vi "Clear Tree.vi"(7 "Tree Refnum In":refnum<vi>, 8 "error in (no error)":errorcluster, 9 "Parent Tag In":string, 10 "Tree":string(tree), 11 "Clear Tree?":bool) -> (0 "error out":errorcluster, 1 "Parent Tag Out":string, 5 "Tree Refnum Out":refnum<vi>)   [LabVIEW 2023]
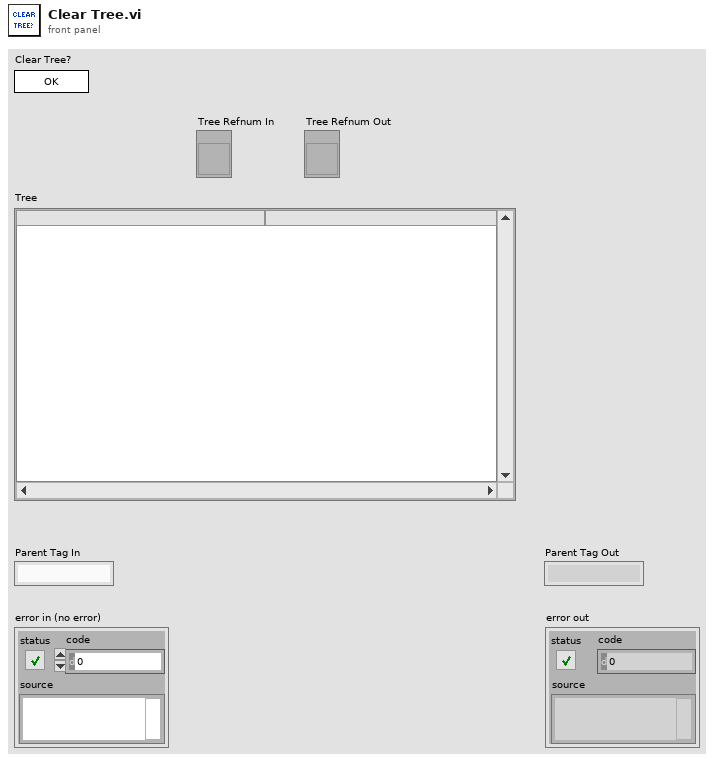
[diagram p1: front panel]
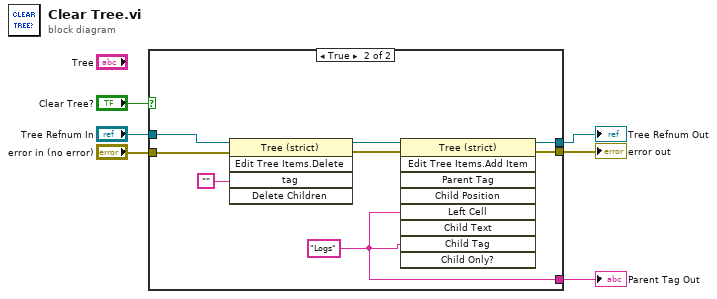
[diagram p0: block diagram]
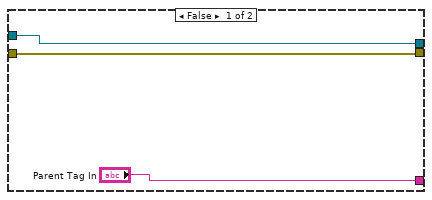
[diagram p2: hidden frame]
diagram:
  n1 = case shown="True" "Clear Tree?" {
    tunnel: [w8 w16] -> w6
    tunnel: [w9 w13] -> w5
    tunnel: "error in (no error)" -> [w8 w12]
    tunnel: "Tree Refnum In" -> [w9 w11]
    tunnel: ["Parent Tag In" w10] -> w1
    frame False {
    }
    frame True {
      w10 = "Logs" ("Parent Tag")
      n2 = invoke class="Tree (strict)" method="Edit Tree Items.Delete"(reference=w11, error in=w12, "tag"="") -> (reference out=w15:refnum<vi>, error out=w17:errorcluster)  [unwired: 2 in, 3 out]
      n3 = invoke on="Invoke Node" class="Tree (strict)" method="Edit Tree Items.Add Item"(reference=w15, error in=w17, "Left Cell"=w10, "Child Tag"=w10) -> (reference out=w13:refnum<vi>, error out=w16:errorcluster)  [unwired: 5 in, 7 out]
    }
  }
  "error out" <- w6
  "Tree Refnum Out" <- w5
  "Parent Tag Out" <- w1
